vi "SetF0Property.vi"(10 "F0":dbl, 11 "props in":T1[](array[typedef])) -> (3 "props out":T1[](array[typedef]))   [LabVIEW 2017, in "McsaDataEventCreator.lvlib"]
uses:
  <vilib>/addons/InsightCM/Devices/Shared/Mcsa/McsaDataEventCreator/McsaDataEventCreator.lvlib
  <vilib>/addons/InsightCM/MessageBus/Base/controls/KeyValuePair.ctl
  <vilib>/addons/InsightCM/Utilities/PropertyHelpers/PropertyHelpers.lvlib
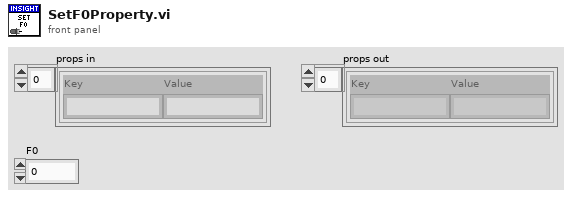
[diagram p1: front panel]
types:
  T1 = typedef "KeyValuePair.ctl" = cluster{"Key":string, "Value":string}
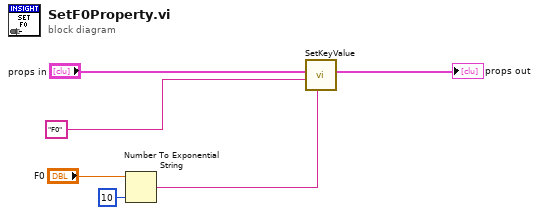
[diagram p0: block diagram]
diagram:
  n1 = Number To Exponential String(number="F0", precision (6)=i16 10) -> (E-format string=w2:string)  [unwired: 2 in]
  n2 = call <vilib>:"SetKeyValue.vi"("value"=w2, "key"="F0", "key value pairs"="props in") -> ("key value pairs out"=→"props out":T1[])  [unwired: 8 in]
